vi "Get array index (Write to JSON)2.vi"(0 "Single element name":string, 5 "previous\n level\n cluster":variant, 7 "JSON first element":bool, 9 "Object name":string, 11 "error in (no error)":errorcluster) -> (4 "index out":i32, 6 "key":string, 8 "VArray":variant, 10 "value":string, 13 "Element Present?":bool, 14 "Array Present?":bool, 15 "error out":errorcluster)   [LabVIEW 2015]
uses:
  <vilib>/regexp/Match Regular Expression.xnode
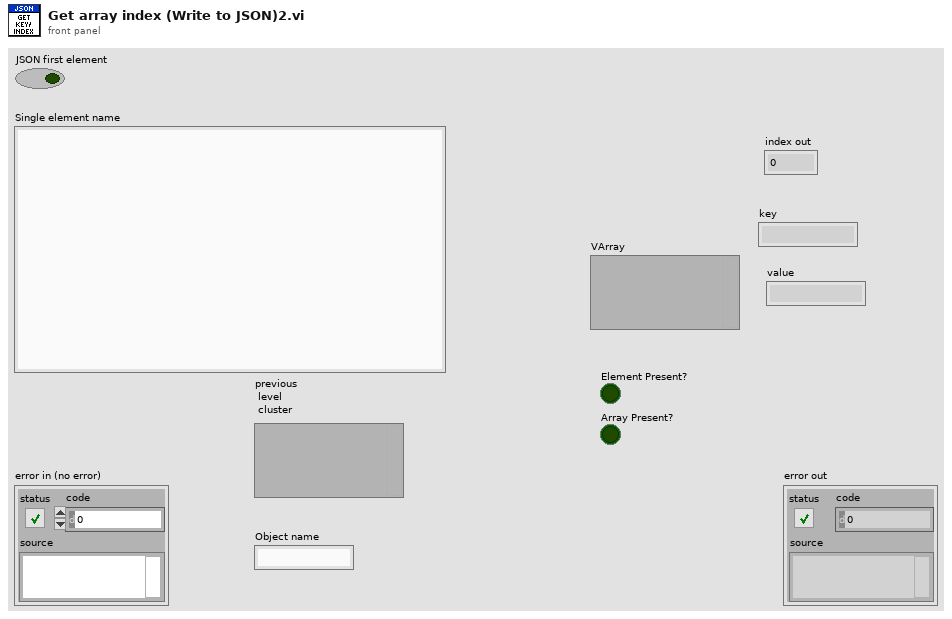
[diagram p1: front panel]
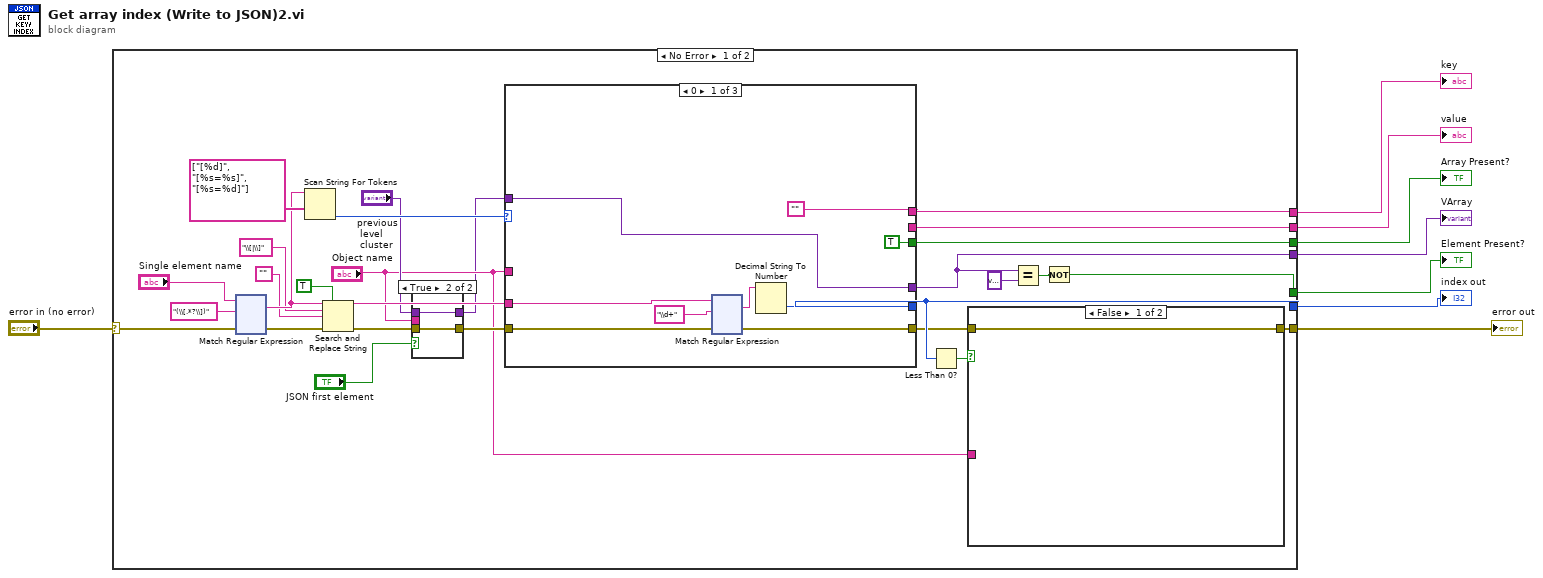
[diagram p0: block diagram]
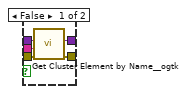
[diagram p2: hidden frame]
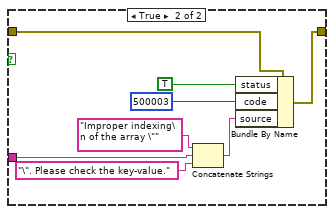
[diagram p3: hidden frame]
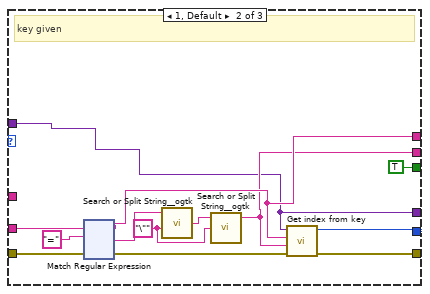
[diagram p4: hidden frame]
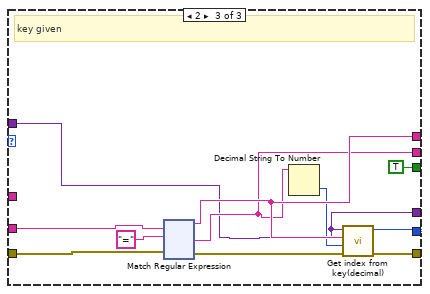
[diagram p5: hidden frame]
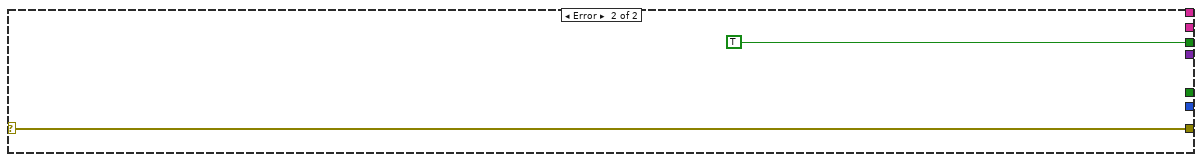
[diagram p6: hidden frame]
diagram:
  n1 = case shown="No Error" "error in (no error)" {
    selector: "error in (no error)" -> [w26 w543]
    tunnel: [w17 w543] -> w7
    tunnel: [w18 _] -> w6
    tunnel: [w25 _] -> w5
    tunnel: [w24 _] -> w4
    tunnel: [w23 TRUE ("found?")] -> w3
    tunnel: [w19 _] -> w2
    tunnel: [w20 _] -> w1
    frame No Error {
      n2 = xnode "Match Regular Expression"("input string"="Single element name", "regular expression"="(\\[.*?\\])", "error in"=w26) -> ("whole match"=w33:string, "error out"=w27:errorcluster)  [unwired: 3 in, 3 out]
      n3 = Scan String For Tokens(7:string[] ["[%d]", "[%s=%s]", "[%s=%d]"] ("operators (none)"), 9:w33) -> (0:w28:i32)  [unwired: 4 in, 3 out]
      n4 = Search and Replace String(replace all?=TRUE ("replace all? (F)"), input string=w33, search string="\\[|\\]", replace string="", error in=w27) -> (result string=w30:string, error out=w14:errorcluster)  [unwired: 3 in, 2 out]
      n5 = case shown="True" "JSON first element" {
        tunnel: w14 -> [w41 w43]
        tunnel: [w40 w43] -> w13
        tunnel: "previous\n level\n cluster" -> [w39 w42]
        tunnel: "Object name" -> [w38 _]
        tunnel: [w37 w42] -> w10
        frame False {
          n6 = call <userlib>:"Get Cluster Element by Name__ogtk.vi"("error in (no error)"=w41, "Element Name"=w38, "Cluster"=w39) -> ("error out"=w40:errorcluster, "VElement"=w37:variant)  [unwired: 6 in, 1 out]
        }
        frame True {
        }
      }
      n7 = case shown="0" w28 {
        tunnel: w30 -> [w61 w188 w313]
        tunnel: w13 -> [w56 w178 w304]
        tunnel: [w58 w187 w311] -> w18
        tunnel: [w53 w176 w310] -> w16
        tunnel: [w57 w186 w309] -> w25
        tunnel: [w57 w179 w308] -> w24
        tunnel: [w55 w177 w303] -> w19
        tunnel: "Object name" -> [_ _ _]
        tunnel: w10 -> [w55 w177 w303]
        tunnel: [TRUE ("found?") TRUE ("found?") TRUE ("found?")] -> w23
        frame 0 {
          w57 = ""
          n8 = xnode "Match Regular Expression"("input string"=w61, "regular expression"="\\d+", "error in"=w56) -> ("whole match"=w59:string, "error out"=w53:errorcluster)  [unwired: 3 in, 3 out]
          n9 = Decimal String To Number(string=w59) -> (number=w58:i32)  [unwired: 2 in, 1 out]
        }
        frame 1, Default {
          w181 = "\"" ("search string/char (-)")
          # "key given"
          n10 = xnode "Match Regular Expression"("input string"=w188, "regular expression"="=", "error in"=w178) -> ("before match"=w186:string, "after match"=w180:string, "error out"=w184:errorcluster)  [unwired: 3 in, 2 out]
          n11 = call <userlib>:"Search or Split String__ogtk.vi"("search string/char (-)"=w181, "string"=w180) -> ("substring after match"=w182:string)  [unwired: 1 in, 2 out]
          n12 = call <userlib>:"Search or Split String__ogtk.vi"("search string/char (-)"=w181, "string"=w182) -> ("substring before match"=w179:string)  [unwired: 1 in, 2 out]
          n13 = call "Get index from key.vi"("error in (no error)"=w184, "value"=w179, "key"=w186, "VElement"=w177) -> ("error out"=w176:errorcluster, "indexOut"=w187:i32)  [unwired: 6 in]
        }
        frame 2 {
          # "key given"
          n14 = xnode "Match Regular Expression"("input string"=w313, "regular expression"="=", "error in"=w304) -> ("before match"=w309:string, "after match"=w308:string, "error out"=w306:errorcluster)  [unwired: 3 in, 2 out]
          n15 = Decimal String To Number(string=w308) -> (number=w307:i32)  [unwired: 2 in, 1 out]
          n16 = call "Get index from key(decimal).vi"("error in (no error)"=w306, "Value(decimal)"=w307, "key"=w309, "VElement"=w303) -> ("error out"=w310:errorcluster, "indexOut"=w311:i32)  [unwired: 6 in]
        }
      }
      n17 = Less Than 0?(x=w18) -> (x < 0?=w15:bool)
      n18 = case shown="False" w15 {
        tunnel: [w44 w49] -> w17
        tunnel: w16 -> [w44 w52]
        tunnel: "Object name" -> [_ w47]
        frame False {
        }
        frame True {
          n19 = Concatenate Strings("Improper indexing\n of the array \"" ("source"), w47, "\". Please check the key-value." ("string")) -> (w45:string)
          n20 = Bundle By Name(cluster=w52, "status"=TRUE, "code"=500003, "source"=w45) -> (w49:errorcluster)
        }
      }
      n21 = Equal?(x=w19, y=variant) -> (x = y?=w21:bool)
      n22 = Not(x=w21) -> (.not. x?=w20:bool)
    }
    frame Error {
    }
  }
  "error out" <- w7
  "index out" <- w6
  "key" <- w5
  "value" <- w4
  "Array Present?" <- w3
  "VArray" <- w2
  "Element Present?" <- w1
